vi "Initialize Acquisition.vi"(8 "error in":errorcluster, 11 "DAQmxChannel":T1) -> (0 "error out":errorcluster, 3 "task out":refnum<k21>)   [LabVIEW 2018]
doc: "Konfiguruje kana³ pomiarowy karty DAQ do pomiaru napiêcia i wyzwala start akwizycji."
uses:
  controls/Daqtypedef.ctl
  <vilib>/DAQmx/create/channels.llb/DAQmx Create Channel (AI-Voltage-Basic).vi
  <vilib>/DAQmx/configure/timing.llb/DAQmx Timing (Sample Clock).vi
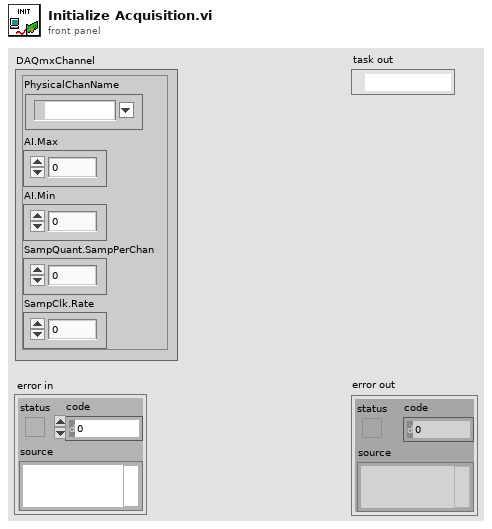
[diagram p1: front panel]
types:
  T1 = typedef "Daqtypedef.ctl" = cluster{"PhysicalChanName":tag, "AI.Max":dbl, "AI.Min":dbl, "SampQuant.SampPerChan":i32, "SampClk.Rate":dbl}
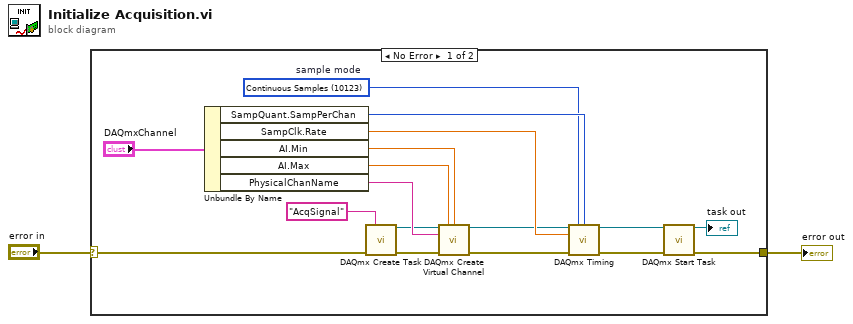
[diagram p0: block diagram]
diagram:
  n1 = case shown="No Error" "error in" {
    selector: "error in" -> [w9 w20]
    tunnel: [w8 w20] -> w2
    frame No Error {
      w13 = 10123 items=["Finite Samples"=10178, "Continuous Samples"=10123, "Hardware Timed Single Point"=12522]  # sample mode
      n2 = Unbundle By Name("DAQmxChannel") -> ("SampQuant.SampPerChan"=w15:i32, "SampClk.Rate"=w14:dbl, "AI.Min"=w18:dbl, "AI.Max"=w17:dbl, "PhysicalChanName"=w16:tag)
      n3 = call <vilib>:"DAQmx Create Task.vi"("new task name"="AcqSignal", "error in"=w9) -> ("task out"=w4:refnum<k21>, "error out"=w5:errorcluster)  [unwired: 12 in]
      n4 = call-poly <vilib>:"DAQmx Create Virtual Channel.vi"("task in"=w4, "maximum value"=w17, "minimum value"=w18, "physical channels"=w16, "error in"=w5) -> ("task out"=w11:refnum<k21>, "error out"=w12:errorcluster)  [unwired: 9 in]
      n5 = call-poly <vilib>:"DAQmx Timing.vi"("task/channels in"=w11, "sample mode"=w13, "samples per channel"=w15, "rate"=w14, "error in"=w12) -> ("task out"=w7:refnum<k21>, "error out"=w10:errorcluster)  [unwired: 9 in]
      n6 = call <vilib>:"DAQmx Start Task.vi"("task/channels in"=w7, "error in"=w10) -> ("task out"=→"task out":refnum<k21>, "error out"=w8:errorcluster)  [unwired: 12 in]
    }
    frame Error {
    }
  }
  "error out" <- w2
